vi "Fetch Measurement (Normal).vi"(6 "Timeout (10000 ms)":i32=10000 min=1, 8 "error in (no error)":errorcluster, 9 "Number of Item (15)":i32=15 min=1 max=255, 10 "Measure Item (1: Plural)":i32(ring)=1 items=["One", "Plural"], 11 "VISA resource name":refnum<visa-resource-name>) -> (0 "error out":errorcluster, 1 "Measurement":dbl[](array[numeric]), 2 "Function":string[](array[string]), 3 "VISA resource name out":refnum<visa-resource-name>)   [LabVIEW 2018, in "Yokogawa WT300 Series.lvlib"]
doc: "Queries the numeric data.\n\n<B>Note:</B> This VI does not check the instrument status. If you want to check the instrument status, call the Error Query VI at the conclusion of the sequence."
uses:
  Yokogawa WT300 Series.lvlib
  Private/Measurement Data Convert (Normal).vi
panel:
  # "ms"
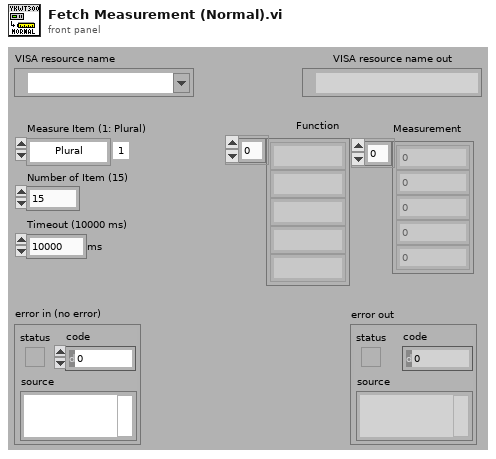
[diagram p1: front panel]
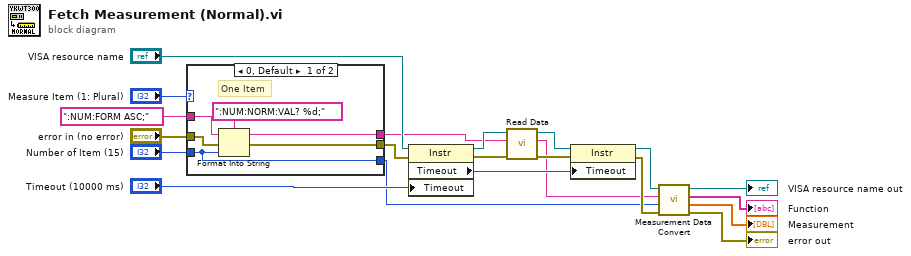
[diagram p0: block diagram]
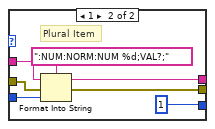
[diagram p2: hidden frame]
diagram:
  n1 = case shown="0, Default" "Measure Item (1: Plural)" {
    tunnel: ":NUM:FORM ASC;" ("形式文字列") -> [w26 w33]
    tunnel: "Number of Item (15)" -> [w22 w32]
    tunnel: "error in (no error)" -> [w25 w31]
    tunnel: [w24 w30] -> w5
    tunnel: [w23 w29] -> w16
    tunnel: [w22 1] -> w11
    frame 0, Default {
      # "One Item"
      n2 = Format Into String(format string=":NUM:NORM:VAL? %d;" ("形式文字列"), initial string=w26, error in=w25, w22) -> (resulting string=w24:string, error out=w23:errorcluster)
    }
    frame 1 {
      # "Plural Item"
      n3 = Format Into String(format string=":NUM:NORM:NUM %d;VAL?;" ("形式文字列"), initial string=w33, error in=w31, w32) -> (resulting string=w30:string, error out=w29:errorcluster)
    }
  }
  n4 = property on="プロパティノード" class="Instr"(reference="VISA resource name", error in=w16, "Timeout"="Timeout (10000 ms)") -> (reference out=w6:refnum<visa-resource-name>, error out=w4:errorcluster, "Timeout"=w15:u32)
  n5 = call "Read Data.vi"("error in (no error)"=w4, "Send Command (Empty)"=w5, "VISA resource name"=w6) -> ("error out"=w2:errorcluster, "Read Data"=w1:string, "VISA resource name out"=w3:refnum<visa-resource-name>)  [unwired: 5 in, 1 out]
  n6 = property on="プロパティノード" class="Instr"(reference=w3, error in=w2, "Timeout"=w15) -> (reference out=w13:refnum<visa-resource-name>, error out=w12:errorcluster)
  n7 = call-poly "Measurement Data Convert.vi"("error in (no error)"=w12, "Item Number Offset (1)"=w11, "Measurement Data (Empty)"=w1, "VISA resource name"=w13) -> ("error out"=→"error out":errorcluster, "Measurement"=→"Measurement":dbl[], "Function"=→"Function":string[], "VISA resource name out"=→"VISA resource name out":refnum<visa-resource-name>)  [unwired: 4 in]
